vi "Write Array.vi"(10 "Array":dbl[](array[numeric]), 11 "Double Array Event in":refnum<class "Double Array Event.lvclass">) -> (3 "Double Array Event out":refnum<class "Double Array Event.lvclass">)   [LabVIEW 2015, in "Example Source.lvlib" / "Double Array Event.lvclass"]
uses:
  Double Array Event.lvclass
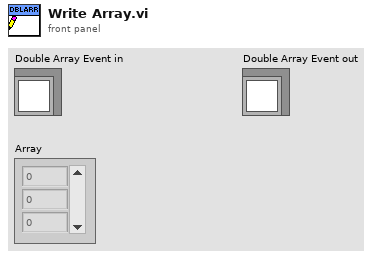
[diagram p1: front panel]
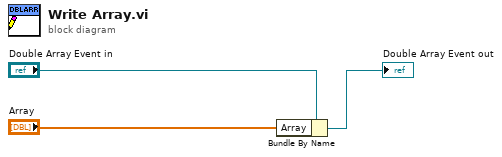
[diagram p0: block diagram]
diagram:
  n1 = Bundle By Name(cluster="Double Array Event in", "Array"="Array") -> (→"Double Array Event out":refnum<class "Double Array Event.lvclass">)
